vi "PEM90_SetWavelength_SetRetardation.vi"() -> ()   [LabVIEW 2016]
panel:
  in  "Read Frecuency":bool
  out "Frecuency":dbl format="%_5f"
  in  "RESET":bool
  in  "Inhibit Retardation":bool
  in  "VISA refnum in":refnum<visa-resource-name>="COM1"
  out "Retardation Out":dbl format="%_3f"
  out "Wavelength Out (nm)":dbl format="%.1f"
  in  "Retardation In":dbl min=0.0 max=19999.900390625 step=0.10000000149011612 format="%.3f"
  in  "Wavelength In (nm)":dbl min=0.0 max=19999.9 step=0.1 format="%.1f"
  out "error out":errorcluster
  in  "error in (no error)":errorcluster
  in  "Stop":bool
  out "Indicator":bool
  out "VISA refnum out":refnum<visa-resource-name>
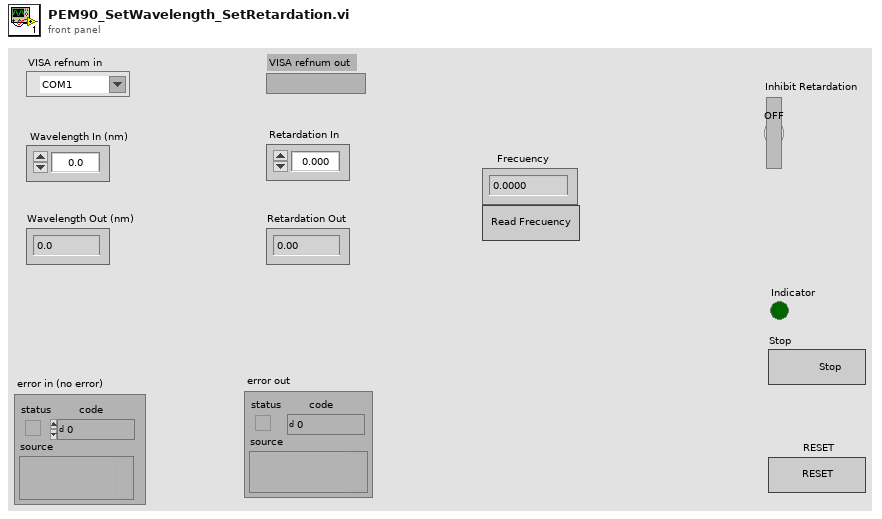
[diagram p1: front panel]
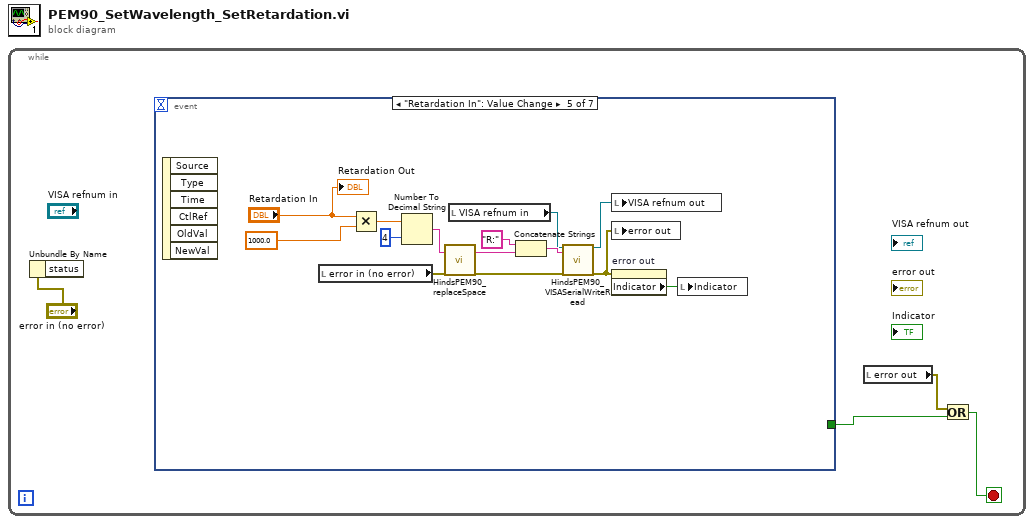
[diagram p0: block diagram]
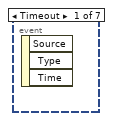
[diagram p2: hidden frame]
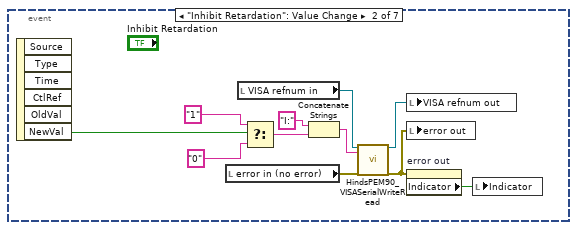
[diagram p3: hidden frame]
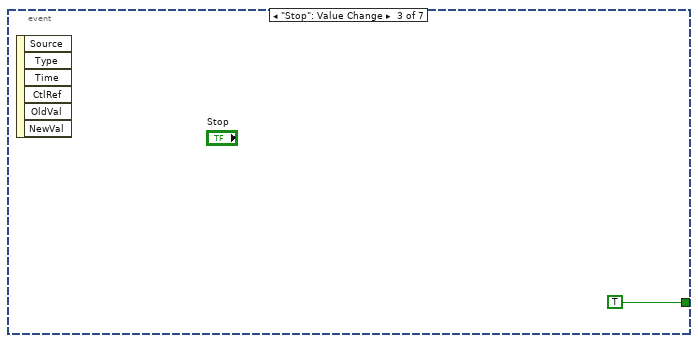
[diagram p4: hidden frame]
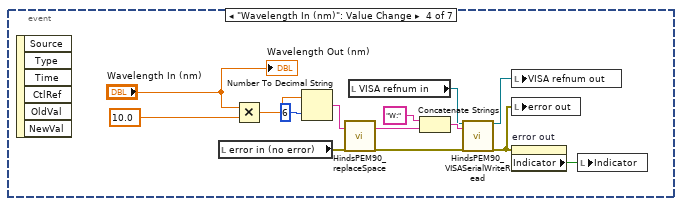
[diagram p5: hidden frame]
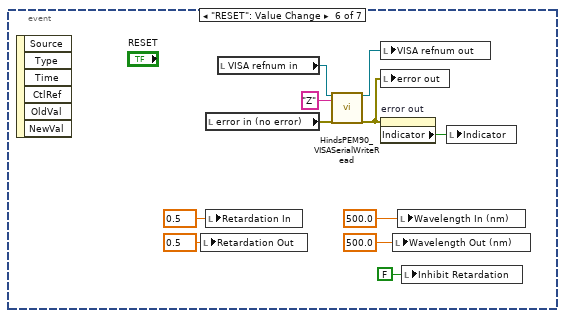
[diagram p6: hidden frame]
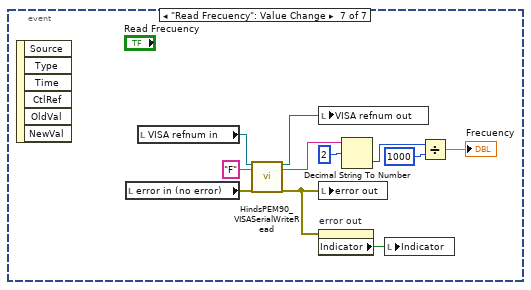
[diagram p7: hidden frame]
diagram:
  n1 = while {
    stop <- w3 stop-if-true
    n2 = Unbundle By Name("error in (no error)") -> ()  [unwired: 1 out]
    n3 = event shown="[4] \"Retardation In\": Value Change" {
      selector: _ -> [_ _ _ _ _ _ _]
      dyn-events: _ -> [_ _ _ _ _ _ _]
      timeout: _ -> [_ _ _ _ _ _ _]
      tunnel: [_ _ TRUE _ _ _ _] -> w1
      event Timeout {
        n4 = event-data() -> ()  [unwired: 1 in, 3 out]
      }
      event "Inhibit Retardation": Value Change {
        n5 = event-data() -> ("NewVal"=w10:bool)  [unwired: 1 in, 5 out]
        n6 = local read "error in (no error)"() -> (w11:errorcluster)
        n7 = local read "VISA refnum in"() -> (w12:refnum<visa-resource-name>)
        n8 = Select(t="1" ("Substring"), s=w10, f="0" ("Substring")) -> (s? t:f=w7:string)
        n9 = Concatenate Strings("I:" ("Substring"), w7) -> (w14:string)
        n10 = call "HindsPEM90_VISASerialWriteRead.vi"("VISA refnum in"=w12, "write"=w14, "error in (no error)"=w11) -> ("VISA refnum out"=w13:refnum<visa-resource-name>, "error out"=w6:errorcluster)  [unwired: 14 in, 1 out]
        n11 = local write "VISA refnum out"(w13) -> ()
        n12 = local write "error out"(w6) -> ()
        n13 = property on="error out" class="Clust (strict)"(error in=w6) -> ("Indicator"=w5:bool)  [unwired: 1 in, 2 out]
        n14 = local write "Indicator"(w5) -> ()
      }
      event "Stop": Value Change {
        n15 = event-data() -> ()  [unwired: 1 in, 6 out]
      }
      event "Wavelength In (nm)": Value Change {
        n16 = event-data() -> ()  [unwired: 1 in, 6 out]
        n17 = local read "error in (no error)"() -> (w20:errorcluster)
        n18 = Multiply(x="Wavelength In (nm)", y=10.0) -> (x*y=w28:dbl)
        n19 = Number To Decimal String(number=w28, width (-)=i16 6) -> (decimal integer string=w23:string)
        n20 = call "HindsPEM90_replaceSpace.vi"("Sting In"=w23, "error in (no error)"=w20) -> ("String Out"=w25:string, "error out"=w24:errorcluster)  [unwired: 16 in]
        n21 = local read "VISA refnum in"() -> (w22:refnum<visa-resource-name>)
        n22 = Concatenate Strings("W:" ("Substring"), w25) -> (w27:string)
        n23 = call "HindsPEM90_VISASerialWriteRead.vi"("VISA refnum in"=w22, "write"=w27, "error in (no error)"=w24) -> ("VISA refnum out"=w21:refnum<visa-resource-name>, "error out"=w17:errorcluster)  [unwired: 14 in, 1 out]
        n24 = local write "VISA refnum out"(w21) -> ()
        n25 = local write "error out"(w17) -> ()
        n26 = property on="error out" class="Clust (strict)"(error in=w17) -> ("Indicator"=w18:bool)  [unwired: 1 in, 2 out]
        n27 = local write "Indicator"(w18) -> ()
        "Wavelength Out (nm)" <- "Wavelength In (nm)"
      }
      event "Retardation In": Value Change {
        n28 = event-data() -> ()  [unwired: 1 in, 6 out]
        n29 = local read "error in (no error)"() -> (w34:errorcluster)
        n30 = Multiply(x="Retardation In", y=1000.0) -> (x*y=w41:dbl)
        n31 = Number To Decimal String(number=w41, width (-)=i16 4) -> (decimal integer string=w40:string)
        n32 = call "HindsPEM90_replaceSpace.vi"("Sting In"=w40, "error in (no error)"=w34) -> ("String Out"=w39:string, "error out"=w44:errorcluster)  [unwired: 16 in]
        n33 = local read "VISA refnum in"() -> (w35:refnum<visa-resource-name>)
        n34 = Concatenate Strings("R:" ("Substring"), w39) -> (w37:string)
        n35 = call "HindsPEM90_VISASerialWriteRead.vi"("VISA refnum in"=w35, "write"=w37, "error in (no error)"=w44) -> ("VISA refnum out"=w36:refnum<visa-resource-name>, "error out"=w32:errorcluster)  [unwired: 14 in, 1 out]
        n36 = local write "VISA refnum out"(w36) -> ()
        n37 = local write "error out"(w32) -> ()
        n38 = property on="error out" class="Clust (strict)"(error in=w32) -> ("Indicator"=w31:bool)  [unwired: 1 in, 2 out]
        n39 = local write "Indicator"(w31) -> ()
        "Retardation Out" <- "Retardation In"
      }
      event "RESET": Value Change {
        n40 = event-data() -> ()  [unwired: 1 in, 6 out]
        n41 = local write "Retardation Out"(0.5 ("Retardation In")) -> ()
        n42 = local read "error in (no error)"() -> (w53:errorcluster)
        n43 = local write "Retardation In"(0.5 ("Retardation In")) -> ()
        n44 = local read "VISA refnum in"() -> (w54:refnum<visa-resource-name>)
        n45 = call "HindsPEM90_VISASerialWriteRead.vi"("VISA refnum in"=w54, "write"="Z" ("Substring"), "error in (no error)"=w53) -> ("VISA refnum out"=w55:refnum<visa-resource-name>, "error out"=w52:errorcluster)  [unwired: 14 in, 1 out]
        n46 = local write "VISA refnum out"(w55) -> ()
        n47 = local write "error out"(w52) -> ()
        n48 = property on="error out" class="Clust (strict)"(error in=w52) -> ("Indicator"=w51:bool)  [unwired: 1 in, 2 out]
        n49 = local write "Wavelength Out (nm)"(500.0 ("Retardation In")) -> ()
        n50 = local write "Wavelength In (nm)"(500.0 ("Retardation In")) -> ()
        n51 = local write "Inhibit Retardation"(FALSE ("Inhibit Retardation")) -> ()
        n52 = local write "Indicator"(w51) -> ()
      }
      event "Read Frecuency": Value Change {
        n53 = event-data() -> ()  [unwired: 1 in, 6 out]
        n54 = local read "error in (no error)"() -> (w64:errorcluster)
        n55 = local read "VISA refnum in"() -> (w65:refnum<visa-resource-name>)
        n56 = call "HindsPEM90_VISASerialWriteRead.vi"("VISA refnum in"=w65, "write"="F" ("Substring"), "error in (no error)"=w64) -> ("VISA refnum out"=w66:refnum<visa-resource-name>, "read buffer"=w60:string, "error out"=w63:errorcluster)  [unwired: 14 in]
        n57 = local write "VISA refnum out"(w66) -> ()
        n58 = local write "error out"(w63) -> ()
        n59 = property on="error out" class="Clust (strict)"(error in=w63) -> ("Indicator"=w62:bool)  [unwired: 1 in, 2 out]
        n60 = Decimal String To Number(string=w60, offset=2) -> (number=w58:i32)  [unwired: 1 in, 1 out]
        n61 = local write "Indicator"(w62) -> ()
        n62 = Divide(x=w58, y=1000) -> (x/y=→"Frecuency":dbl)
      }
    }
    n63 = local read "error out"() -> (w2:errorcluster)
    n64 = Or(x=w2, y=w1) -> (x .or. y?=w3:bool)
  }
